vi "FOLI double.vi"(0 "Array":dbl[](array[numeric]), 2 "Array size":i32, 7 "Numeric":dbl) -> (4 "Array out":dbl[](array[numeric]))   [LabVIEW 2014]
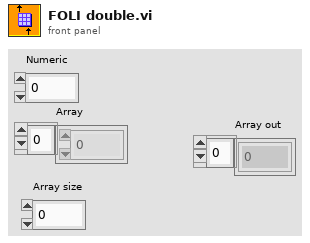
[diagram p1: front panel]
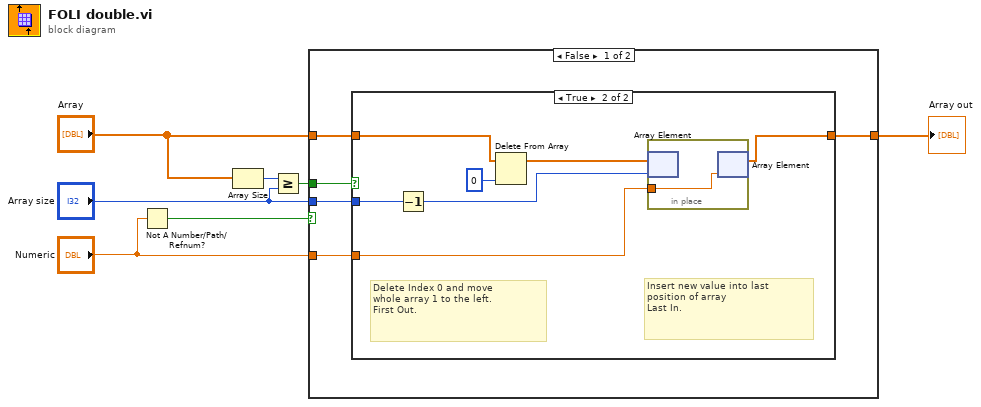
[diagram p0: block diagram]
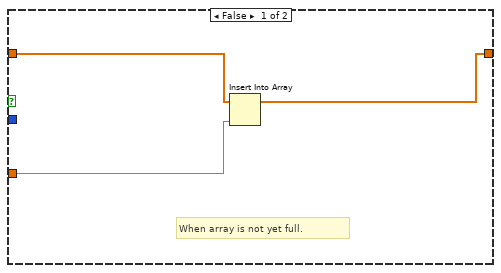
[diagram p2: hidden frame]
diagram:
  n1 = Not A Number/Path/Refnum?(number/path/refnum="Numeric") -> (NaN/Path/Refnum?=w2:bool)
  n2 = Array Size(array="Array") -> (size(s)=w7:i32)
  n3 = Greater Or Equal?(x=w7, y="Array size") -> (x >= y?=w6:bool)
  n4 = case shown="False" w2 {
    tunnel: w6 -> [w12 _]
    tunnel: "Array" -> [w11 w24]
    tunnel: "Numeric" -> [w10 _]
    tunnel: [w9 w24] -> w4
    tunnel: "Array size" -> [w8 _]
    frame False {
      n5 = case shown="True" w12 {
        tunnel: [w13 w16] -> w9
        tunnel: w11 -> [w14 w21]
        tunnel: w10 -> [w15 w17]
        tunnel: w8 -> [_ w20]
        frame False {
          # "When array is not yet full."
          n6 = Insert Into Array(array=w14, new element=w15) -> (w13:dbl[])  [unwired: 1 in]
        }
        frame True {
          # "Insert new value into last\nposition of array\nLast In."
          # "Delete Index 0 and move \nwhole array 1 to the left.\nFirst Out."
          n7 = Decrement(x=w20) -> (x-1=w18:i32)
          n8 = Delete From Array(array=w21, index=0) -> (array with subset deleted=w19:dbl[])  [unwired: 1 in, 1 out]
          n9 = in-place {
            in-place-border: w17 -> [w23]
            n10 = in-place-array #1(w19, w18) -> ()  [unwired: 1 out]
            n11 = in-place-array #1(w23) -> (w16:dbl[])  [unwired: 1 out]
          }
        }
      }
    }
    frame True {
      # "String is empty."
    }
  }
  "Array out" <- w4
